vi "Configure Math.vi"(0 "VISA resource name":refnum<visa-resource-name>, 1 "Degree Value (20.0)":dbl=20.0 format="%_3g", 2 "Upper Limit (0.00)":dbl format="%_3g", 3 "Lower Limit (0.00)":dbl format="%_3g", 5 "Operation (13:None)":T1(ring)=enum."None", 7 "Scale Value (1.00)":dbl=1.0 format="%_3g", 9 "Percent Value (1.00%)":dbl=1.0 format="%_3g", 11 "error in (no error)":errorcluster, 12 "dB Reference Point (1.00 dB)":dbl=1.0 format="%_3g", 13 "dBm Resistance (50 Ohms)":dbl=50.0 format="%_3g", 14 "Null Offset (0.00)":dbl format="%_3g") -> (4 "VISA resource name out":refnum<visa-resource-name>, 15 "error out":errorcluster)   [LabVIEW 2010, in "Agilent 3458.lvlib"]
doc: "Configures the DMM for math operations. When measurements are taken, the selected math operation is applied to each measurement taken. Note that the results for the HI/LO test can only retrieved using the Query Questionable Data Register VI."
uses:
  <instrlib>/Agilent 3458/Agilent 3458.lvlib
panel:
  # "DB Measurements"
  # "Limit"
  # "Null Function"
  # "Scale Function"
  # "Percent Function"
  # "Degree Function"
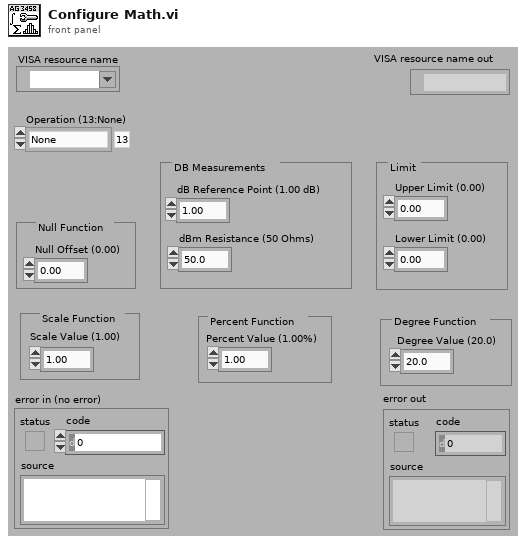
[diagram p1: front panel]
types:
  T1 = enum16{"CRTD85", "CRTD92", "CTHRM", "CTHRM2K", "CTHRM10K", "dB", "dBm", "Filter", "FRTD85", "FRTD92", "FTHRM", "FTHRM2K", "FTHRM10K", "None", "Null", "Pass/Fail", "Percent", "RMS", "Scale", "Statistics"}
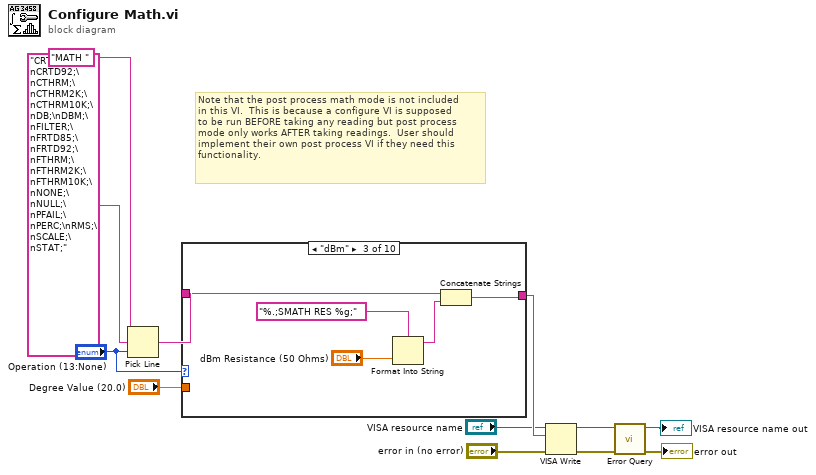
[diagram p0: block diagram]
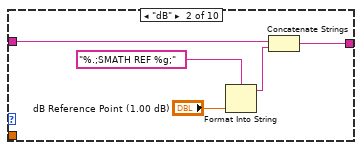
[diagram p3: hidden frame]
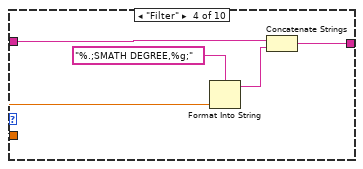
[diagram p4: hidden frame]
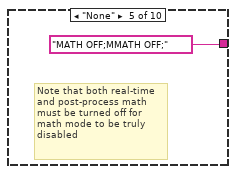
[diagram p5: hidden frame]
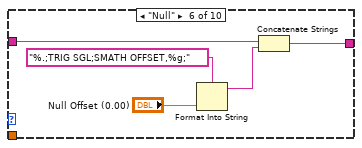
[diagram p6: hidden frame]
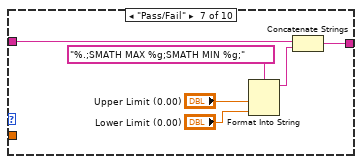
[diagram p7: hidden frame]
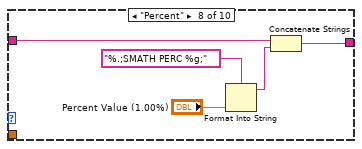
[diagram p8: hidden frame]
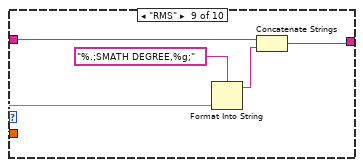
[diagram p9: hidden frame]
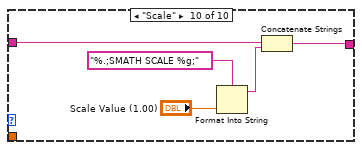
[diagram p10: hidden frame]
diagram:
  # "Note that the post process math mode is not included\nin this VI.  This is because a configure VI is supposed\nto be run BEFORE taking any reading but post process \nmode only works AFTER taking readings.  User should\nimplement their own post process VI if they need this\nfunctionality."
  n1 = Pick Line(string ("")="MATH ", multi-line string="CRTD85;\nCRTD92;\nCTHRM;\nCTHRM2K;\nCTHRM10K;\nDB;\nDBM;\nFILTER;\nFRTD85;\nFRTD92;\nFTHRM;\nFTHRM2K;\nFTHRM10K;\nNONE;\nNULL;\nPFAIL;\nPERC;\nRMS;\nSCALE;\nSTAT;", line index="Operation (13:None)") -> (output string=w9:string)
  n2 = case shown="\"dBm\"" "Operation (13:None)" {
    tunnel: w9 -> [w13 w17 w21 w25 _ w33 w39 w44 w48 w53]
    tunnel: [w13 w15 w20 w27 "MATH OFF;MMATH OFF;" w31 w38 w42 w47 w52] -> w7
    tunnel: "Degree Value (20.0)" -> [_ _ _ w24 _ _ _ _ w46 _]
    frame Default {
    }
    frame "dB" {
      n3 = Format Into String(format string="%.;SMATH REF %g;", "dB Reference Point (1.00 dB)") -> (resulting string=w16:string)  [unwired: 2 in, 1 out]
      n4 = Concatenate Strings(w17, w16) -> (w15:string)
    }
    frame "dBm" {
      n5 = Format Into String(format string="%.;SMATH RES %g;", "dBm Resistance (50 Ohms)") -> (resulting string=w22:string)  [unwired: 2 in, 1 out]
      n6 = Concatenate Strings(w21, w22) -> (w20:string)
    }
    frame "Filter" {
      n7 = Format Into String(format string="%.;SMATH DEGREE,%g;", w24) -> (resulting string=w26:string)  [unwired: 2 in, 1 out]
      n8 = Concatenate Strings(w25, w26) -> (w27:string)
    }
    frame "None" {
      # "Note that both real-time\nand post-process math \nmust be turned off for\nmath mode to be truly\ndisabled"
    }
    frame "Null" {
      n9 = Format Into String(format string="%.;TRIG SGL;SMATH OFFSET,%g;", "Null Offset (0.00)") -> (resulting string=w32:string)  [unwired: 2 in, 1 out]
      n10 = Concatenate Strings(w33, w32) -> (w31:string)
    }
    frame "Pass/Fail" {
      n11 = Format Into String(format string="%.;SMATH MAX %g;SMATH MIN %g;", "Upper Limit (0.00)", "Lower Limit (0.00)") -> (resulting string=w36:string)  [unwired: 2 in, 1 out]
      n12 = Concatenate Strings(w39, w36) -> (w38:string)
    }
    frame "Percent" {
      n13 = Format Into String(format string="%.;SMATH PERC %g;", "Percent Value (1.00%)") -> (resulting string=w43:string)  [unwired: 2 in, 1 out]
      n14 = Concatenate Strings(w44, w43) -> (w42:string)
    }
    frame "RMS" {
      n15 = Format Into String(format string="%.;SMATH DEGREE,%g;", w46) -> (resulting string=w49:string)  [unwired: 2 in, 1 out]
      n16 = Concatenate Strings(w48, w49) -> (w47:string)
    }
    frame "Scale" {
      n17 = Format Into String(format string="%.;SMATH SCALE %g;", "Scale Value (1.00)") -> (resulting string=w54:string)  [unwired: 2 in, 1 out]
      n18 = Concatenate Strings(w53, w54) -> (w52:string)
    }
  }
  n19 = VISA Write(VISA resource name="VISA resource name", write buffer=w7, error in (no error)="error in (no error)") -> (VISA resource name out=w11:refnum<visa-resource-name>, error out=w10:errorcluster)  [unwired: 1 out]
  n20 = call <instrlib>:"Error Query.vi"("error in (no error)"=w10, "VISA resource name"=w11) -> ("error out"=→"error out":errorcluster, "VISA resource name out"=→"VISA resource name out":refnum<visa-resource-name>)  [unwired: 6 in, 2 out]
